vi "Init Control.vi"(5 "Group":refnum<class "Group.lvclass">, 7 "VolatusAPI":refnum<class "VolatusAPI.lvclass">, 8 "error in (no error)":errorcluster, 9 "Control MsgQ":refnum<class "MessageQ.lvclass">, 10 "Config Element":refnum<class "Config Element.lvclass">, 11 "Valve in":refnum<class "MultiControl.lvclass">) -> (0 "error out":errorcluster, 3 "Valve out":refnum<class "MultiControl.lvclass">)   [LabVIEW 2020, in "VolatusControl.lvlib" / "MultiControl.lvclass"]
uses:
  MultiControl.lvclass
  lv-cdm/CDM-Config/Config Element/Config Element.lvclass
  Volatus/VolatusAPI/VolatusAPI.lvclass
  Volatus/MessageQ/MessageQ.lvclass
  lv-vecto/Vecto/Group/Group.lvclass
  C:/dev/lv20CE/relink/lv-vecto/Vecto/GroupAbstract/GroupAbstract.lvclass
  <vilib>/Utility/miscctls.llb/LVMapReplaceAction.ctl
  MultiControl.lvclass/MultiControl.ctl
  lv-vecto/Vecto/GroupAbstract/GroupAbstract.lvclass
  lv-vecto/Vecto/Vecto.lvlib
  C:/dev/lv20CE/relink/lv-vecto/Vecto/Group/Group.lvclass
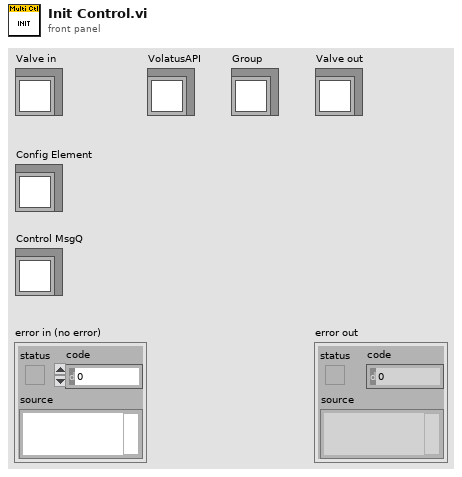
[diagram p1: front panel]
types:
  T1 = typedef "LVMapReplaceAction.ctl" = enum32{"Modify Entry only if found", "Add or Modify Entry", "Delete Entry"}
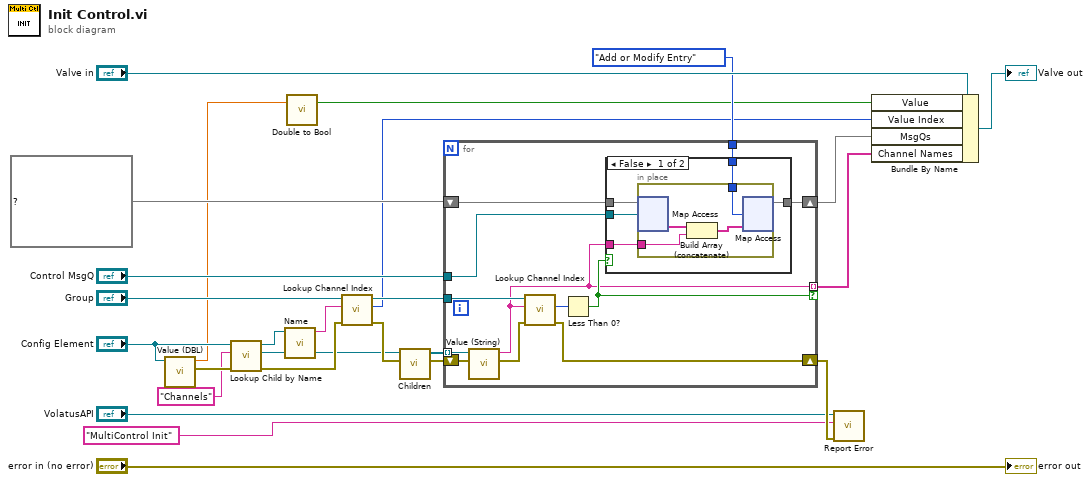
[diagram p0: block diagram]
diagram:
  n1 = call "Value (DBL).vi"("Config Element in"="Config Element") -> ("error out"=w24:errorcluster, "DBL Value"=w6:dbl)  [unwired: 9 in]
  n2 = call "Lookup Child by Name.vi"("error in (no error)"=w24, "Name"="Channels", "Config Element in"="Config Element") -> ("error out"=w25:errorcluster, "Child"=w19:refnum<class "Config Element.lvclass">, "Config Element out"=w4:refnum<class "Config Element.lvclass">)  [unwired: 5 in, 1 out]
  n3 = call "Name.vi"("Config Element in"=w4) -> ("Name"=w2:string)  [unwired: 9 in, 1 out]
  n4 = call "Double to Bool.vi"("Double"=w6) -> ("Bool"=w5:bool)  [unwired: 2 in]
  n5 = call "Lookup Channel Index.vi"("error in (no error)"=w25, "Channel Name"=w2, "GroupAbstract in"="Group") -> ("error out"=w26:errorcluster, "Index"=w1:i32, "GroupAbstract out"=w3:refnum<class "Group.lvclass">)  [unwired: 6 in]
  n6 = call "Children.vi"("error in (no error)"=w26, "Config Element in"=w19) -> ("error out"=w14:errorcluster, "Elements"=w18:refnum<class "Config Element.lvclass">[])  [unwired: 8 in]
  n7 = for {
    tunnel: w18 -> [w38] mode=indexing
    shift-right: [w27] -> w23
    shift-left: w14 -> [w37]
    shift-right: [w31] -> w8
    shift-left: map{refnum<class "MessageQ.lvclass">, string[]} {} ("MsgQs") -> [w32]
    tunnel: "Control MsgQ" -> [w30]
    tunnel: w3 -> [w36]
    tunnel: [w29] -> w9 mode=indexing if=w33
    tunnel: LVMapReplaceAction."Add or Modify Entry" ("action") -> [w28]
    n8 = call "Value (String).vi"("error in (no error)"=w37, "Config Element in"=w38) -> ("error out"=w35:errorcluster, "String Value"=w29:string)  [unwired: 8 in]
    n9 = call "Lookup Channel Index.vi"("error in (no error)"=w35, "Channel Name"=w29, "GroupAbstract in"=w36) -> ("error out"=w27:errorcluster, "Index"=w34:i32)  [unwired: 6 in, 1 out]
    n10 = Less Than 0?(x=w34) -> (x < 0?=w33:bool)
    n11 = case shown="False" w33 {
      tunnel: w32 -> [w43 w48]
      tunnel: [w39 w48] -> w31
      tunnel: w30 -> [w42 _]
      tunnel: w29 -> [w41 _]
      tunnel: w28 -> [w40 _]
      frame False {
        n12 = in-place {
          in-place-border: w41 -> [w46]
          in-place-border: w40 -> [w44]
          n13 = in-place-map #1(w43, w42) -> (w47:string[])  [unwired: 1 in, 1 out]
          n14 = Build Array (concatenate)(w47, w46) -> (w45:string[])
          n15 = in-place-map #1(w45, w44) -> (w39:map{refnum<class "MessageQ.lvclass">, string[]})  [unwired: 2 out]
        }
      }
      frame True {
      }
    }
  }
  n16 = call "Report Error.vi"("error in (no error)"=w23, "Context"="MultiControl Init", "VolatusAPI in"="VolatusAPI") -> ()  [unwired: 7 in, 2 out]
  n17 = Bundle By Name(cluster="Valve in", "Value"=w5, "Value Index"=w1, "MsgQs"=w8, "Channel Names"=w9) -> (→"Valve out":refnum<class "MultiControl.lvclass">)
  "error out" <- "error in (no error)"
